vi "STS_Get_Meas_Power_Rawdata.vi"(8 "错误输入（无错误）":errorcluster, 10 "setting":refnum<k24>, 11 ".NET引用句柄输入":refnum<k24>) -> (0 "error out":errorcluster, 1 "powerdata":sgl[](array[numeric]), 3 "引用输出":refnum<k24>)   [LabVIEW 2017]
doc: "monitor data is 1 data for each sweep. It can be overwrite."
uses:
  D:/test/ILSTS/LV_IL/LV_IL_Sample_x64/DLL/STSProcess.dll
  DLL/STSProcess.dll
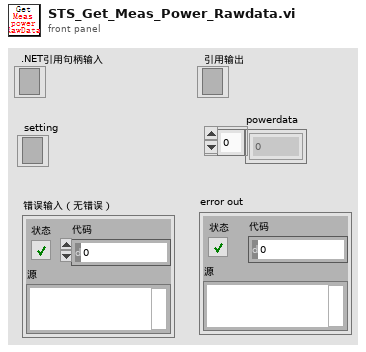
[diagram p1: front panel]
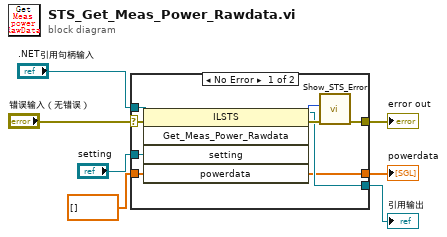
[diagram p0: block diagram]
diagram:
  n1 = case shown="No Error" "错误输入（无错误）" {
    selector: "错误输入（无错误）" -> [w15 w19]
    tunnel: ".NET引用句柄输入" -> [w16 w18]
    tunnel: [w12 w19] -> w5
    tunnel: [w11 w18] -> w4
    tunnel: "setting" -> [w10 _]
    tunnel: sgl[] [] ("powerdata") -> [w9 w17]
    tunnel: [w8 w17] -> w1
    frame No Error {
      n2 = invoke class="ILSTS" method="Get_Meas_Power_Rawdata"(reference=w16, error in=w15, "setting"=w10, "powerdata"=w9) -> (reference out=w11:refnum<k24>, error out=w14:errorcluster, "Get_Meas_Power_Rawdata"=w13:i32, "powerdata"=w8:sgl[])  [unwired: 1 in, 1 out]
      n3 = call "Show_STS_Error.vi"("error in (no error)"=w14, "Error"=w13) -> ("error out"=w12:errorcluster)  [unwired: 9 in]
    }
    frame Error {
    }
  }
  "error out" <- w5
  "引用输出" <- w4
  "powerdata" <- w1
